vi "Autonomous.vi"() -> ()   [LabVIEW 2018]
panel:
  in  "Autonomous":T1(ring)
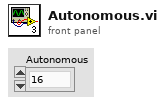
[diagram p1: front panel]
types:
  T1 = enum16{"16", "15", "14", "13", "12", "11", "10", "9", "8", "7", "6", "5", "4", "3", "2", "1"}
  T2 = enum16{"N/A", "Hatch Panel Zone 1", "Hatch Panel Zone 2", "Hatch Panel Zone 3", "Cargo Zone 1", "Cargo Zone 2", "Cargo Zone 3"}
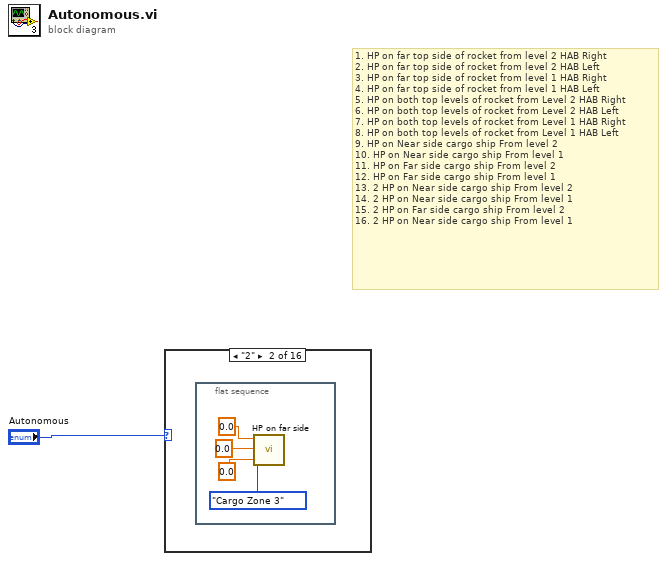
[diagram p0: block diagram]
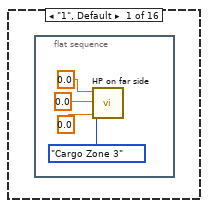
[diagram p2: hidden frame]
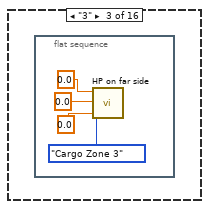
[diagram p3: hidden frame]
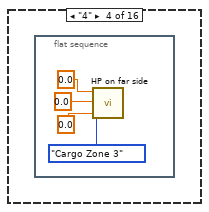
[diagram p4: hidden frame]
diagram:
  # "1. HP on far top side of rocket from level 2 HAB Right\n2. HP on far top side of rocket from level 2 HAB Left\n3. HP on far top side of rocket from level 1 HAB Right\n4. HP on far top side of rocket from level 1 HAB Left\n5. HP on both top levels of rocket from Level 2 HAB Right\n6. HP on both top levels of rocket from Level 2 HAB Left\n7. HP on both top levels of rocket from Level 1 HAB Right\n8. HP on both top levels of rocket from Level 1 HAB Left\n9. HP on Near side cargo ship From level 2\n10. HP on Near side cargo ship From level 1\n11. HP on Far side cargo ship From level 2\n12. HP on Far side cargo ship From level 1\n13. 2 HP on Near side cargo ship From level 2\n14. 2 HP on Near side cargo ship From level 1\n15. 2 HP on Far side cargo ship From level 2\n16. 2 HP on Near side cargo ship From level 1"
  n1 = case shown="\"2\"" "Autonomous" {
    frame "1", Default {
      n2 = flat-sequence {
        frame #0 {
          n3 = call "HP on far side.vi"("LiftLocation"=T2."Cargo Zone 3", "Z"=0.0, "Y"=0.0, "X"=0.0) -> ()  [unwired: 8 in]
        }
      }
    }
    frame "2" {
      n4 = flat-sequence {
        frame #0 {
          n5 = call "HP on far side.vi"("LiftLocation"=T2."Cargo Zone 3", "Z"=0.0, "Y"=0.0, "X"=0.0) -> ()  [unwired: 8 in]
        }
      }
    }
    frame "3" {
      n6 = flat-sequence {
        frame #0 {
          n7 = call "HP on far side.vi"("LiftLocation"=T2."Cargo Zone 3", "Z"=0.0, "Y"=0.0, "X"=0.0) -> ()  [unwired: 8 in]
        }
      }
    }
    frame "4" {
      n8 = flat-sequence {
        frame #0 {
          n9 = call "HP on far side.vi"("LiftLocation"=T2."Cargo Zone 3", "Z"=0.0, "Y"=0.0, "X"=0.0) -> ()  [unwired: 8 in]
        }
      }
    }
    frame "5" {
    }
    frame "6" {
    }
    frame "7" {
    }
    frame "8" {
    }
    frame "9" {
    }
    frame "10" {
    }
    frame "11" {
    }
    frame "12" {
    }
    frame "13" {
    }
    frame "14" {
    }
    frame "15" {
    }
    frame "16" {
    }
  }
